vi "main - Copy.vi"() -> ()   [LabVIEW 2019]
panel:
  out "pal detected":bool
  in  "pal num":string
  in  "Stop (F)":bool
  out "Image Out":T1(plugin-control)
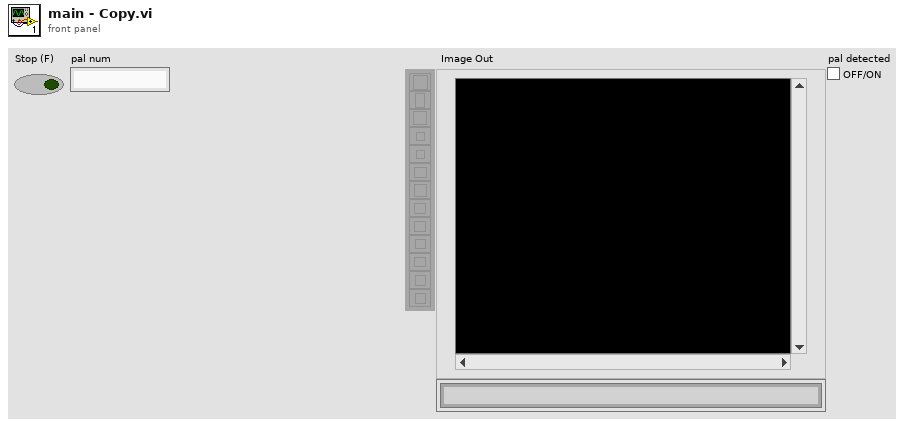
[diagram p1: front panel]
types:
  T1 = typedef "IMAQ Image.ctl" = refnum<image>
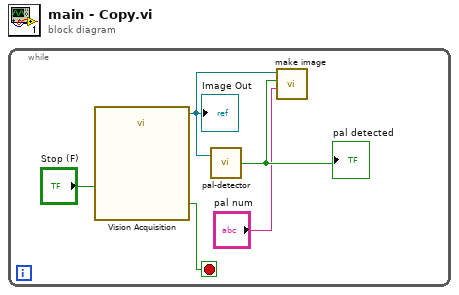
[diagram p0: block diagram]
diagram:
  n1 = while {
    stop <- w4 stop-if-true
    n2 = call "Vision Acquisition"("Stop (F)"="Stop (F)") -> ("Image Out"=w2:T1, "Stopped"=w4:bool)  [unwired: 24 in, 1 out]
    "Image Out" <- w2
    n3 = call "pal-detector.vi"("Image"=w2) -> ("pal detected"=w3:bool)  [unwired: 1 in]
    "pal detected" <- w3
    n4 = call "make image.vi"("pal num"="pal num", "take a photo"=w3, "Image"=w2) -> ()  [unwired: 1 in, 1 out]
  }
